vi "AlliGator Phasor Plot Image Cursor Location to Phasor v2.vi"(8 "Error In":errorcluster, 9 "Phasor Plot Size":T1={"H"=512, "V"=512, "Margin"=0.2}, 11 "Coords in":T2) -> (0 "Error Out":errorcluster, 3 "Phasor":T3)   [LabVIEW 2021, in "AlliGator Phasor Plot.lvlib"]
doc: "Converts Phasor Plot Image cursor location to Phasor value."
uses:
  Phasor/Phasor (g, s).ctl
  <vilib>/Utility/miscctls.llb/LVPoint32TypeDef.ctl
  AlliGator Phasor Plot Size.ctl
  AlliGator Phasor Plot.lvlib
  Phasor/Phasor.lvlib
panel:
  # "see the AlliGator License on the block diagram (Ctrl+E or Window:Show Block Diagram)"
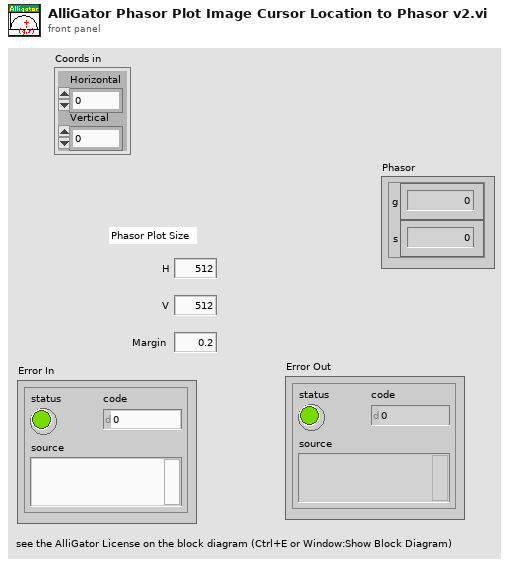
[diagram p1: front panel]
types:
  T1 = typedef "AlliGator Phasor Plot.lvlib/AlliGator Phasor Plot Size.ctl" = cluster{"H":i32, "V":i32, "Margin":dbl}
  T2 = typedef "LVPoint32TypeDef.ctl" = cluster{"Horizontal":i32, "Vertical":i32}
  T3 = typedef "Phasor.lvlib/Phasor (g, s).ctl" = cluster{"g":dbl, "s":dbl}
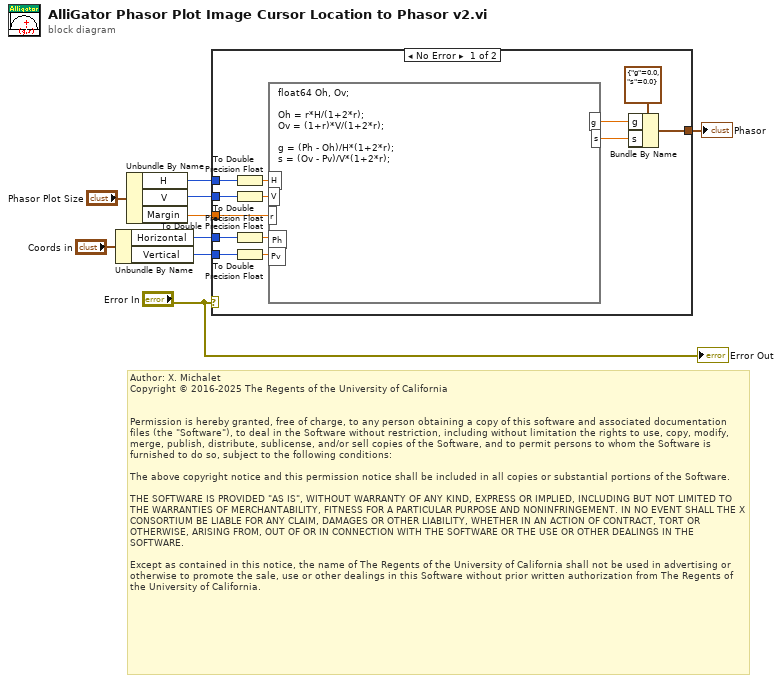
[diagram p0: block diagram]
diagram:
  # "Author: X. Michalet\nCopyright © 2016-2025 The Regents of the University of California\n \n\nPermission is hereby granted, free of charge, to any person obtaining a copy of this software and associated documentation files (the \"Software\"), to deal in the Software without restriction, including without limitation the rights to use, copy, modify, merge, publish, distribute, sublicense, and/or sell copies of the Software, and to permit persons to whom the Software is furnished to do so, subject to the following conditions:\n\nThe above copyright notice and this permission notice shall be included in all copies or substantial portions of the Software.\n\nTHE SOFTWARE IS PROVIDED \"AS IS\", WITHOUT WARRANTY OF ANY KIND, EXPRESS OR IMPLIED, INCLUDING BUT NOT LIMITED TO THE WARRANTIES OF MERCHANTABILITY, FITNESS FOR A PARTICULAR PURPOSE AND NONINFRINGEMENT. IN NO EVENT SHALL THE X CONSORTIUM BE LIABLE FOR ANY CLAIM, DAMAGES OR OTHER LIABILITY, WHETHER IN AN ACTION OF CONTRACT, TORT OR OTHERWISE, ARISING FROM, OUT OF OR IN CONNECTION WITH THE SOFTWARE OR THE USE OR OTHER DEALINGS IN THE SOFTWARE.\n\nExcept as contained in this notice, the name of The Regents of the University of California shall not be used in advertising or otherwise to promote the sale, use or other dealings in this Software without prior written authorization from The Regents of the University of California."
  n1 = Unbundle By Name("Coords in") -> ("Horizontal"=w4:i32, "Vertical"=w3:i32)
  n2 = Unbundle By Name("Phasor Plot Size") -> ("H"=w6:i32, "V"=w7:i32, "Margin"=w8:dbl)
  n3 = case shown="No Error" "Error In" {
    tunnel: w8 -> [w22 _]
    tunnel: w7 -> [w21 _]
    tunnel: w6 -> [w20 _]
    tunnel: w4 -> [w19 _]
    tunnel: w3 -> [w18 _]
    tunnel: [w15 _] -> w2
    frame No Error {
      n4 = To Double Precision Float(number=w20) -> (double precision float=w13:dbl)
      n5 = To Double Precision Float(number=w21) -> (double precision float=w12:dbl)
      n6 = To Double Precision Float(number=w19) -> (double precision float=w11:dbl)
      n7 = To Double Precision Float(number=w18) -> (double precision float=w10:dbl)
      n8 = formula code="float64 Oh, Ov;\n\nOh = r*H/(1+2*r);\nOv = (1+r)*V/(1+2*r);\n\ng = (Ph - Oh)/H*(1+2*r);\ns = (Ov - Pv)/V*(1+2*r);"("H"=w13, "V"=w12, "r"=w22, "Ph"=w11, "Pv"=w10) -> ("g"=w17:dbl, "s"=w16:dbl)
      n9 = Bundle By Name(cluster=T3 {"g"=0.0, "s"=0.0} ("Phasor"), "g"=w17, "s"=w16) -> (w15:T3)
    }
    frame Error {
    }
  }
  "Phasor" <- w2
  "Error Out" <- "Error In"
